vi "dKing.vi"(1 "boardGroup":i32[][](array[numeric]), 2 "turn":i32) -> (0 "isDKing":bool)   [LabVIEW 2024]
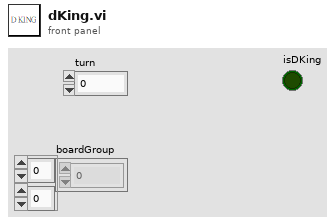
[diagram p1: front panel]
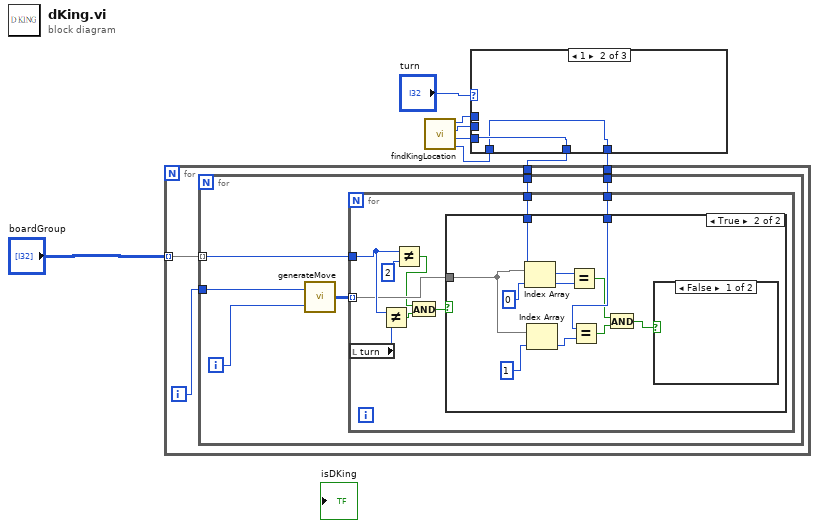
[diagram p0: block diagram]
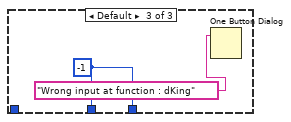
[diagram p3: hidden frame]
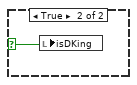
[diagram p5: hidden frame]
diagram:
  n1 = call "findKingLocation.vi"() -> ("bj"=w4:i32, "bi"=w5:i32, "rj"=w6:i32, "ri"=w7:i32)
  n2 = case shown="1" "turn" {
    tunnel: w7 -> [w10 _ _]
    tunnel: w6 -> [w9 _ _]
    tunnel: w5 -> [_ w12 _]
    tunnel: w4 -> [_ w11 _]
    tunnel: [w10 w12 w13] -> w3
    tunnel: [w9 w11 w13] -> w2
    frame 0 {
    }
    frame 1 {
    }
    frame Default {
      w13 = -1 ("bi")
      n3 = One Button Dialog(message="Wrong input at function : dKing") -> ()  [unwired: 1 in, 1 out]
    }
  }
  n4 = for {
    tunnel: "boardGroup" -> [w17] mode=indexing
    tunnel: w3 -> [w16]
    tunnel: w2 -> [w15]
    i -> [w18]
    n5 = for {
      tunnel: w18 -> [w24]
      tunnel: w17 -> [w21] mode=indexing
      tunnel: w16 -> [w20]
      tunnel: w15 -> [w19]
      i -> [w23]
      n6 = call "generateMove.vi"("j"=w23, "i"=w24) -> ("Array"=w22:i32[][])
      n7 = for {
        tunnel: w22 -> [w30] mode=indexing
        tunnel: w21 -> [w32]
        tunnel: w20 -> [w29]
        tunnel: w19 -> [w28]
        n8 = local read "turn"() -> (w31:i32)
        n9 = Not Equal?(x=w32, y=w31) -> (x != y?=w26:bool)
        n10 = Not Equal?(x=w32, y=2) -> (x != y?=w27:bool)
        n11 = And(x=w27, y=w26) -> (x .and. y?=w25:bool)
        n12 = case shown="True" w25 {
          tunnel: w30 -> [_ w42]
          tunnel: w29 -> [_ w40]
          tunnel: w28 -> [_ w38]
          frame False {
          }
          frame True {
            n13 = Index Array(array=w42, index=0) -> (element=w39:i32)
            n14 = Index Array(array=w42, index=1) -> (element=w37:i32)
            n15 = Equal?(x=w40, y=w39) -> (x = y?=w36:bool)
            n16 = Equal?(x=w38, y=w37) -> (x = y?=w35:bool)
            n17 = And(x=w36, y=w35) -> (x .and. y?=w34:bool)
            n18 = case shown="False" w34 {
              selector: w34 -> [_ w44]
              frame False {
              }
              frame True {
                n19 = local write "isDKing"(w44) -> ()
              }
            }
          }
        }
      }
    }
  }
